vi "TMDS.RemoveQuotesFromPath.vi"(8 "error in (no error)":errorcluster, 11 "Data":path) -> (0 "error out":errorcluster, 3 "Path":path)   [LabVIEW 2014, in "NIAnalysis.lvlib"]
uses:
  NIAnalysis.lvlib
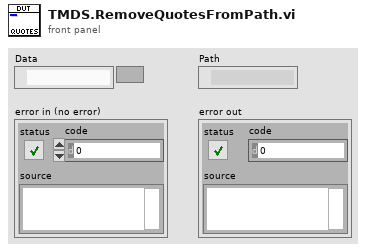
[diagram p1: front panel]
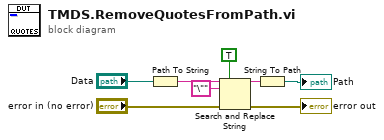
[diagram p0: block diagram]
diagram:
  n1 = Path To String(path="Data") -> (string=w7:string)
  n2 = Search and Replace String(replace all?=TRUE ("replace all? (F)"), input string=w7, search string="\"", error in="error in (no error)") -> (result string=w8:string, error out=→"error out":errorcluster)  [unwired: 4 in, 2 out]
  n3 = String To Path(string=w8) -> (path=→"Path":path)
